vi "onAttributeOverwrite.vi"(8 "Current Attribute":refnum<class "Attribute.lvclass">, 10 "New Attribute":refnum<class "Attribute.lvclass">) -> (2 "Attribute out":refnum<class "Attribute.lvclass">)   [LabVIEW 2013, in "Attribute.lvclass"]
uses:
  Attribute.lvclass
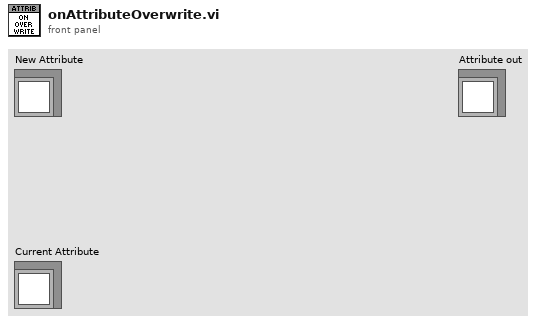
[diagram p1: front panel]
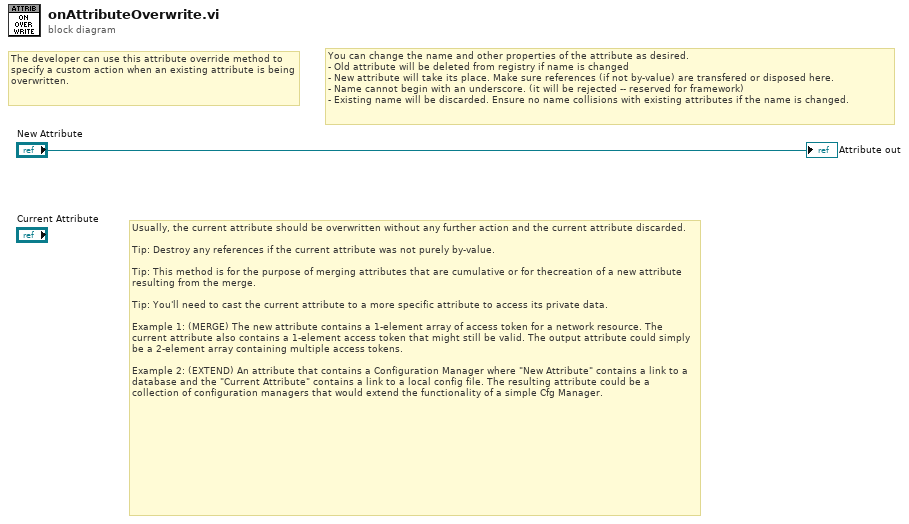
[diagram p0: block diagram]
diagram:
  # "You can change the name and other properties of the attribute as desired.\n- Old attribute will be deleted from registry if name is changed\n- New attribute will take its place. Make sure references (if not by-value) are transfered or disposed here.\n- Name cannot begin with an underscore. (it will be rejected -- reserved for framework)\n- Existing name will be discarded. Ensure no name collisions with existing attributes if the name is changed."
  # "Usually, the current attribute should be overwritten without any further action and the current attribute discarded.\n\nTip: Destroy any references if the current attribute was not purely by-value.\n\nTip: This method is for the purpose of merging attributes that are cumulative or for thecreation of a new attribute resulting from the merge. \n\nTip: You'll need to cast the current attribute to a more specific attribute to access its private data.\n\nExample 1: (MERGE) The new attribute contains a 1-element array of access token for a network resource. The current attribute also contains a 1-element access token that might still be valid. The output attribute could simply be a 2-element array containing multiple access tokens.\n\nExample 2: (EXTEND) An attribute that contains a Configuration Manager where \"New Attribute\" contains a link to a database and the \"Current Attribute\" contains a link to a local config file. The resulting attribute could be a collection of configuration managers that would extend the functionality of a simple Cfg Manager."
  # "The developer can use this attribute override method to specify a custom action when an existing attribute is being overwritten."
  "Attribute out" <- "New Attribute"
